vi "CAN convert.vi"(0 "MSG  array":T1(array[cluster])) -> (1 "CAN":i32[](array[numeric]), 2 "Overload":bool[](array[boolean]))   [LabVIEW 2011]
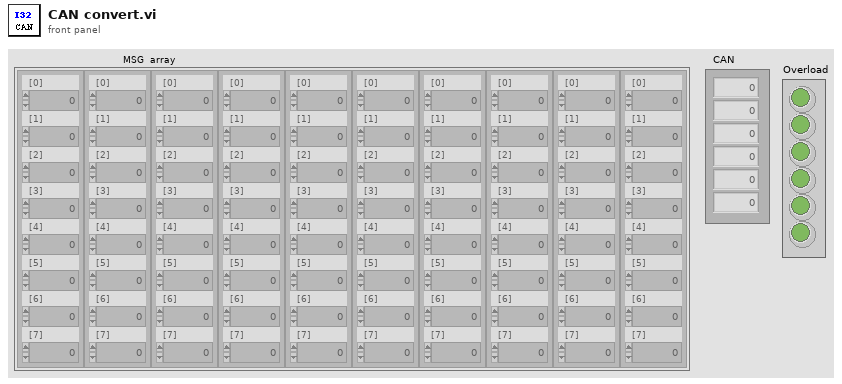
[diagram p1: front panel]
types:
  T1 = cluster{"[0]":u8, "[1]":u8, "[2]":u8, "[3]":u8, "[4]":u8, "[5]":u8, "[6]":u8, "[7]":u8}[]
  T2 = cluster{"[0]":u8, "[1]":u8, "[2]":u8, "[3]":u8, "[4]":u8, "[5]":u8, "[6]":u8, "[7]":u8}
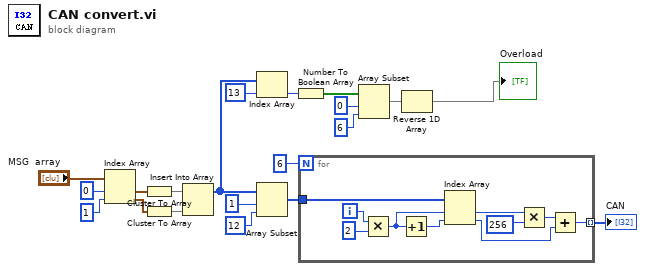
[diagram p0: block diagram]
diagram:
  n1 = Index Array(array="MSG  array", index #1=0 ("인덱스"), index #2=1 ("인덱스")) -> (element #1=w13:T2, element #2=w12:T2)
  n2 = Cluster To Array(cluster=w13) -> (array=w14:u8[])
  n3 = Cluster To Array(cluster=w12) -> (array=w15:u8[])
  n4 = Insert Into Array(array=w14, new element=w15) -> (w8:u8[])  [unwired: 1 in]
  n5 = Index Array(array=w8, index=13 ("인덱스")) -> (element=w6:u8)
  n6 = Array Subset(array=w8, index=1 ("인덱스"), length=12 ("길이")) -> (w19:u8[])
  n7 = Number To Boolean Array(number=w6) -> (Boolean array=w5:bool[])
  n8 = for {
    N: 6 -> [_]
    tunnel: w19 -> [w26]
    tunnel: [w21] -> w9 mode=indexing
    i -> [w30]
    n9 = Multiply(x=w30, y=2) -> (x*y=w27:i32)
    n10 = Increment(x=w27) -> (x+1=w28:i32)
    n11 = Index Array(array=w26, index #1=w27, index #2=w28) -> (element #1=w25:u8, element #2=w23:u8)
    n12 = Multiply(x=w25, y=256) -> (x*y=w22:i32)
    n13 = Add(x=w22, y=w23) -> (x+y=w21:i32)
  }
  "CAN" <- w9
  n14 = Array Subset(array=w5, index=0 ("인덱스"), length=6 ("길이")) -> (w2:bool[])
  n15 = Reverse 1D Array(array=w2) -> (reversed array=→"Overload":bool[])
